vi "Set Current.vi"(8 "error in (no error)":errorcluster, 9 "Pins":string[](array[string]), 10 "current level":dbl format="%.6p", 11 "Semiconductor Module Context":T1) -> (0 "error out":errorcluster, 3 "Semiconductor Module Context Out":T1)   [LabVIEW 2013]
uses:
  <vilib>/NI_TestStand_SemiconductorModule/NI_TestStand_Semiconductor_Module.lvlibp/PinMap/General/SemiconductorModuleContext.ctl
  <instrlib>/niDCPower/nidcpower.llb/niDCPower Wait For Event - Event.ctl
  <vilib>/NI_TestStand_SemiconductorModule/NI_TestStand_Semiconductor_Module.lvlibp/PinMap/DC Power/PinsToNIDCPowerSessions.vi
  <vilib>/NI_TestStand_SemiconductorModule/NI_TestStand_Semiconductor_Module.lvlibp
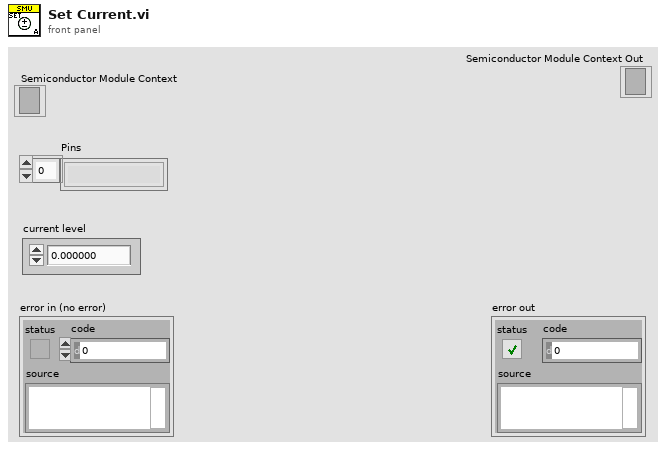
[diagram p1: front panel]
types:
  T1 = typedef "NI_TestStand_Semiconductor_Module.lvlibp/SemiconductorModuleContext.ctl" = refnum<k7>
  T2 = typedef "niDCPower Wait For Event - Event.ctl" = i32
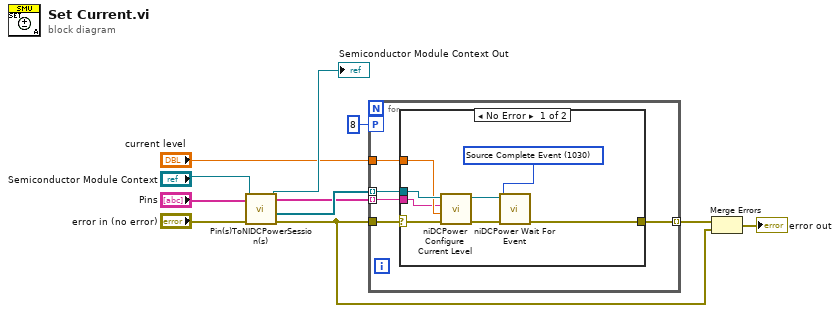
[diagram p0: block diagram]
diagram:
  n1 = call-poly <vilib>:"Pin(s)ToNIDCPowerSession(s).vi"("error in (no error)"="error in (no error)", "Pins"="Pins", "Semiconductor Module Context"="Semiconductor Module Context") -> ("error out"=w7:errorcluster, "Instrument Sessions"=w11:refnum<k15>[], "Channel Lists"=w10:string[], "Semiconductor Module Context Out"=→"Semiconductor Module Context Out":T1)  [unwired: 4 in, 1 out]
  n2 = for {
    tunnel: w11 -> [w16] mode=indexing
    tunnel: w10 -> [w15] mode=indexing
    tunnel: w7 -> [w14]
    tunnel: [w13] -> w8 mode=indexing
    workers-P: 8 -> [_]
    tunnel: "current level" -> [w12]
    n3 = case shown="No Error" w14 {
      selector: w14 -> [w19 w25]
      tunnel: [w17 w25] -> w13
      tunnel: w16 -> [w21 _]
      tunnel: w15 -> [w18 _]
      tunnel: w12 -> [w20 _]
      frame No Error {
        w24 = T2 1030 items=["Source Complete Event"=1030, "Measure Complete Event"=1031, "Sequence Iteration Complete Event"=1032, "Sequence Engine Done Event"=1033, "Pulse Complete Event"=1051, "Ready For Pulse Trigger Event"=1052] ("event")
        n4 = call <instrlib>:"niDCPower Configure Current Level.vi"("error in (no error)"=w19, "current level"=w20, "channel name"=w18, "instrument handle"=w21) -> ("error out"=w23:errorcluster, "instrument handle out"=w22:refnum<k15>)  [unwired: 6 in]
        n5 = call <instrlib>:"niDCPower Wait For Event.vi"("error in (no error)"=w23, "event"=w24, "instrument handle"=w22) -> ("error out"=w17:errorcluster)  [unwired: 7 in, 1 out]
      }
      frame Error {
      }
    }
  }
  n6 = Merge Errors(w8, w7) -> (→"error out":errorcluster)
